vi "reactor_merge.vi"(10 "reactor_path":path) -> ()   [LabVIEW 2019]
uses:
  lib/libSimulationControl/libSimulationControl.lvlib
  lib/libFileFunctions/libFileFunctions.lvlib
panel:
  # "*******************************************************************\nBiogas Plant Control\n\nAuthor: Paul Zügel\nGCSC-Frankfurt am Main 2020\n\n*******************************************************************"
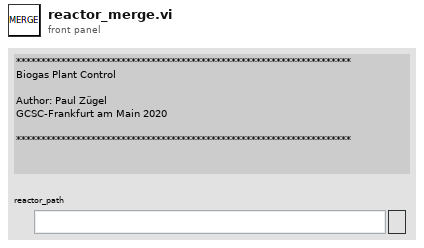
[diagram p1: front panel]
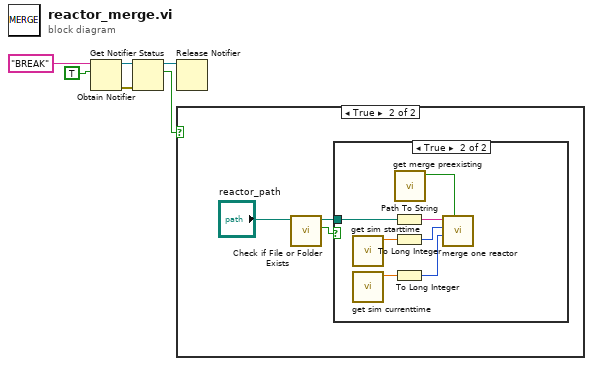
[diagram p0: block diagram]
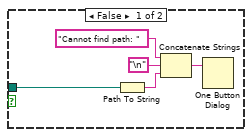
[diagram p3: hidden frame]
diagram:
  n1 = Obtain Notifier(name (unnamed)="BREAK", notification data type=TRUE) -> (notifier out=w4:refnum<notifier>, error out=w3:errorcluster)  [unwired: 2 in, 1 out]
  n2 = Get Notifier Status(notifier=w4, error in (no error)=w3) -> (notifier out=w1:refnum<notifier>, current notification=w2:bool)  [unwired: 3 out]
  n3 = Release Notifier(notifier=w1) -> ()  [unwired: 2 in, 3 out]
  n4 = case shown="True" w2 {
    frame False {
    }
    frame True {
      n5 = call <vilib>:"Check if File or Folder Exists.vi"("path"="reactor_path") -> ("file or folder exists?"=w8:bool, "dup path"=w7:path)  [unwired: 8 in, 1 out]
      n6 = case shown="True" w8 {
        tunnel: w7 -> [w14 w16]
        frame False {
          n7 = Path To String(path=w14) -> (string=w12:string)
          n8 = Concatenate Strings("Cannot find path: " ("string"), "\n", w12) -> (w10:string)
          n9 = One Button Dialog(message=w10) -> ()  [unwired: 1 in, 1 out]
        }
        frame True {
          n10 = call "get sim starttime.vi"() -> ("sim_starttime"=w20:dbl)  [unwired: 10 in, 1 out]
          n11 = call "get sim currenttime.vi"() -> ("current_time"=w21:dbl)  [unwired: 10 in, 1 out]
          n12 = Path To String(path=w16) -> (string=w19:string)
          n13 = To Long Integer(number=w20) -> (32bit integer=w18:i32)
          n14 = To Long Integer(number=w21) -> (32bit integer=w17:i32)
          n15 = call "get merge preexisting.vi"() -> ("function return"=w15:bool)  [unwired: 10 in, 1 out]
          n16 = call "merge one reactor.vi"("merge_preexisting"=w15, "current_starttime"=w17, "simulation_starttime"=w18, "working_dir"=w19) -> ()  [unwired: 7 in, 1 out]
        }
      }
    }
  }
